vi "Do.vi"(8 "error in (no error)":errorcluster, 10 "Actor in":refnum<class "Actor.lvclass">, 11 "RequestShutdownMsg":refnum<class "RequestShutdownMsg.lvclass">) -> (0 "error out":errorcluster, 2 "Actor out":refnum<class "Actor.lvclass">)   [LabVIEW 2026, in "Lumberjack.lvlib" / "RequestShutdownMsg.lvclass"]
doc: "Start the shutdown flush fence on the manager. Hands the manager its own enqueuer (carried in this message as managerEnqueuer, supplied by Logger.Shutdown) to BeginFlushDrain, which seeds selfEnqueuer, sends a FlushAppenderMsg to every registered appender, and sets pendingFlushCount. Actor: LogManager (SRS-LMBR-002)."
uses:
  RequestShutdownMsg.lvclass
  <vilib>/ActorFramework/Actor/Actor.lvclass
  LogManager/LogManager.lvclass/LogManager.lvclass
  C:/Program Files (x86)/National Instruments/LabVIEW 2026/vi.lib/ActorFramework/Actor/Actor.lvclass
  RequestShutdownMsg.lvclass/RequestShutdownMsg.ctl
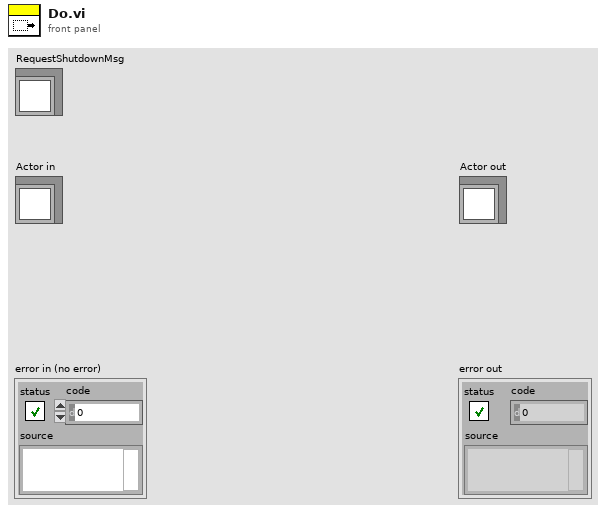
[diagram p1: front panel]
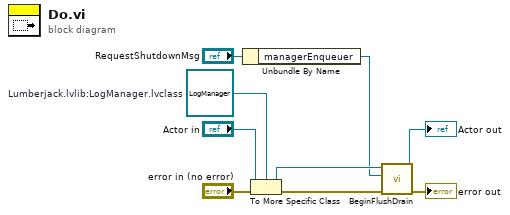
[diagram p0: block diagram]
diagram:
  w2 = refnum<class "LogManager.lvclass"> refnum  # Lumberjack.lvlib:LogManager.lvclass
  n1 = Unbundle By Name("RequestShutdownMsg") -> ("managerEnqueuer"=w3:refnum<class "Message Enqueuer.lvclass">)
  n2 = To More Specific Class(target class=w2, reference="Actor in", error in="error in (no error)") -> (specific class reference=w4:refnum<class "LogManager.lvclass">, error out=w7:errorcluster)
  n3 = call "BeginFlushDrain.vi"("error in (no error)"=w7, "managerEnqueuer"=w3, "LogManager in"=w4) -> ("error out"=→"error out":errorcluster, "LogManager out"=→"Actor out":refnum<class "LogManager.lvclass">)  [unwired: 7 in]
